vi "TurnAngleOperationOpenLoop.vi"(7 "RobotDriveRef in":T1={"RobotDriveDevRef"={"DevStatus"={"status"=FALSE, "code"=0, "source"=""}, "Motors[]"=[], "Square Inputs"=FALSE, "Max Output"=0.0}, "Control Mode"=enum."Percent VBus", "Motor Settings"={"Wheel Radius"=0.0, "Encoder Ticks Per Rev"=0.0, "Gear Ratio"=0.0, "ClimbRev"=0.0}, "Default Control Mode"=enum."Unchanged / Invalid", "Speed Mag"=0.0}, 8 "error in (no error)":errorcluster, 9 "SubSystem Data":T10, 10 "Control Mode":T8, 11 "Command Loop Data":cluster{"Start Time (ms)":u32, "Iterations":i32}) -> (0 "error out":errorcluster, 1 "Left Motor Value":dbl, 2 "RobotDriveRef out":T1={"RobotDriveDevRef"={"DevStatus"={"status"=FALSE, "code"=0, "source"=""}, "Motors[]"=[], "Square Inputs"=FALSE, "Max Output"=0.0}, "Control Mode"=enum."Percent VBus", "Motor Settings"={"Wheel Radius"=0.0, "Encoder Ticks Per Rev"=0.0, "Gear Ratio"=0.0, "ClimbRev"=0.0}, "Default Control Mode"=enum."Unchanged / Invalid", "Speed Mag"=0.0}, 3 "Wait Time":dbl, 4 "Waveform Chart":cluster{"Angle To Turn out":dbl, "Yaw":dbl}(graph), 5 "Finished":bool, 6 "Right Motor Value":dbl)   [LabVIEW 2015]
uses:
  Drive Setpoints.ctl
  Drive Operations.ctl
  Advanced Drive VIs/RobotDrive Type Def.ctl
  <vilib>/Rock Robotics/WPI/MotorControl/WPI_MotorControlDeviceRef.ctl
  <vilib>/Rock Robotics/WPI/MotorControl/WPI_MotorControlType.ctl
  <vilib>/Rock Robotics/SystemInterfaces/DIO/FPGA_DIOPWMChannel.ctl
  <vilib>/Rock Robotics/WPI/PWM/WPI_PWMDeadband.ctl
  <vilib>/Rock Robotics/WPI/CAN/Jaguar/SubVIs/WPI_CANJaguar_ControlMode.ctl
  <vilib>/Rock Robotics/WPI/CAN/TalonSRX/WPI_CANTalonSRX_APIControlMode.ctl
  Advanced Drive VIs/Drive Motor Settings.ctl
  NavX/NavX Global.vi
  NavX/Library/navX Library v2.lvlib
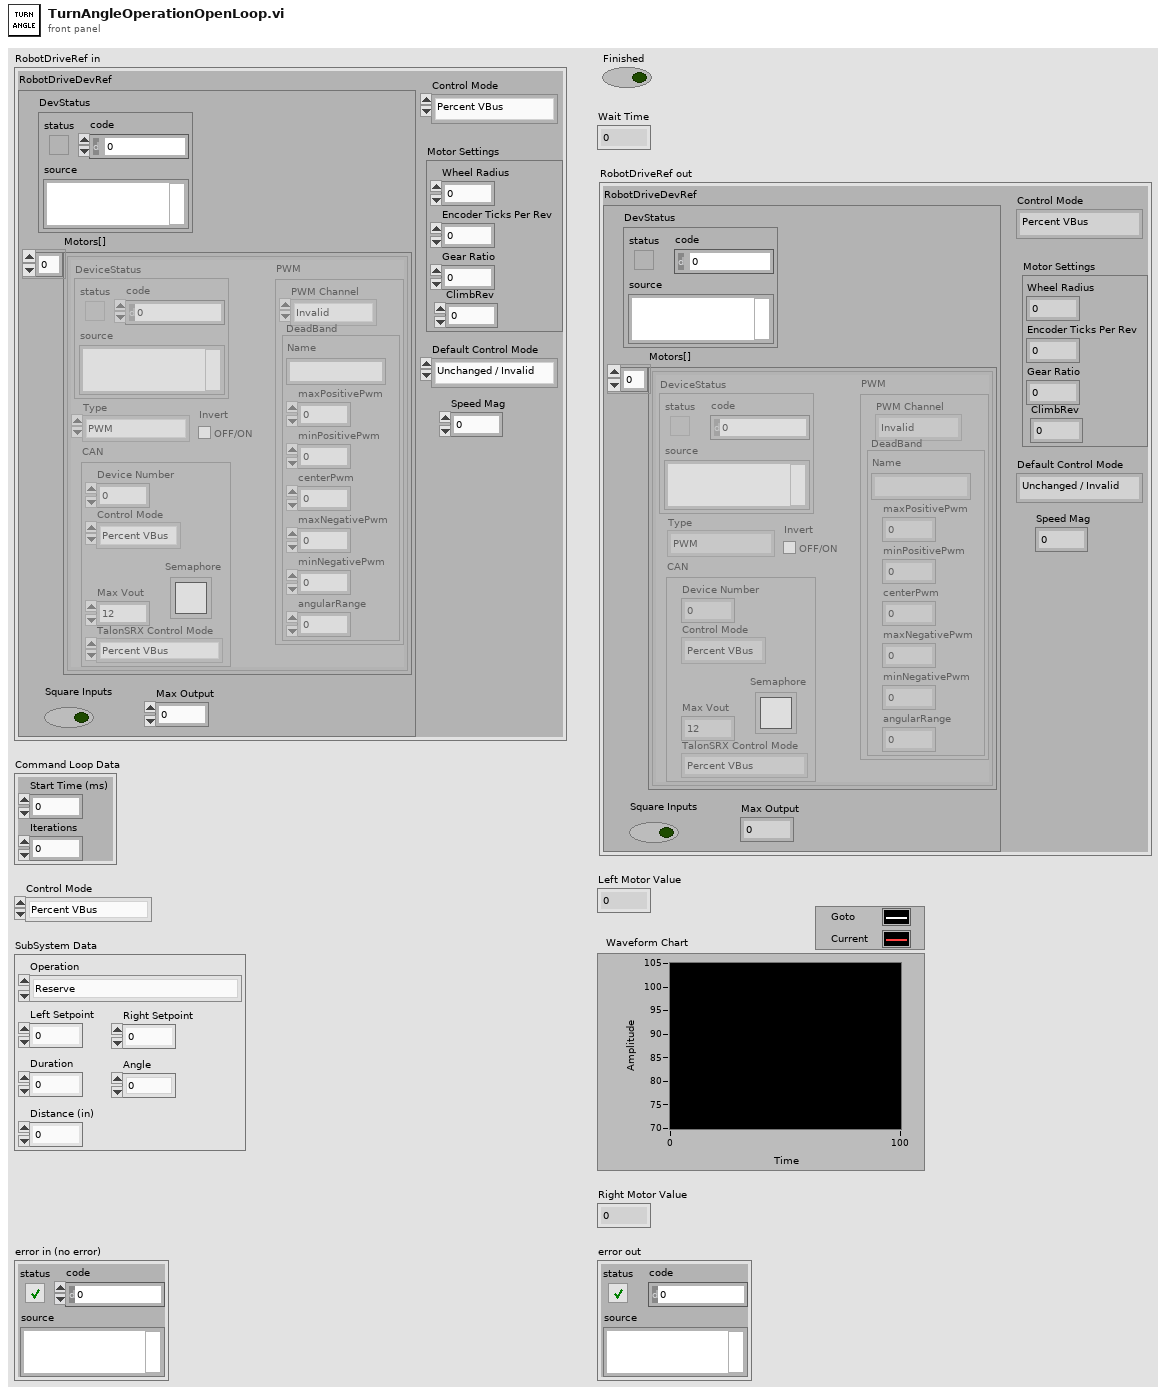
[diagram p1: front panel]
types:
  T1 = typedef "RobotDrive Type Def.ctl" = cluster{"RobotDriveDevRef":cluster{"DevStatus":errorcluster, "Motors[]":T2[], "Square Inputs":bool, "Max Output":dbl}, "Control Mode":T8, "Motor Settings":T9, "Default Control Mode":T8, "Speed Mag":dbl}
  T2 = typedef "WPI_MotorControlDeviceRef.ctl" = cluster{"DeviceStatus":errorcluster, "Type":T3, "PWM":cluster{"PWM Channel":T4, "DeadBand":T5}, "CAN":cluster{"Device Number":u8, "Control Mode":T6, "Semaphore":T7, "Max Vout":dbl, "TalonSRX Control Mode":T8}, "Invert":bool}
  T3 = typedef "WPI_MotorControlType.ctl" = enum16{"PWM", "CAN", "CANTalonSRX"}
  T4 = typedef "FPGA_DIOPWMChannel.ctl" = enum8{"PWM 0", "PWM 1", "PWM 2", "PWM 3", "PWM 4", "PWM 5", "PWM 6", "PWM 7", "PWM 8", "PWM 9", "PWM MXP 0", "PWM MXP 1", "PWM MXP 2", "PWM MXP 3", "PWM MXP 4", "PWM MXP 5", "PWM MXP 6", "PWM MXP 7", "PWM MXP 8", "PWM MXP 9", "Invalid"}
  T5 = typedef "WPI_PWMDeadband.ctl" = cluster{"Name":string, "maxPositivePwm":i32, "minPositivePwm":i32, "centerPwm":i32, "maxNegativePwm":i32, "minNegativePwm":i32, "angularRange":u16}
  T6 = typedef "WPI_CANJaguar_ControlMode.ctl" = enum8{"Percent VBus", "Current", "Speed", "Position", "Voltage"}
  T7 = typedef "Semaphore RefNum" = refnum<k1>
  T8 = typedef "WPI_CANTalonSRX_APIControlMode.ctl" = enum8{"Percent VBus", "Speed", "Position", "Slave", "Unchanged / Invalid", "Voltage Compensation", "Current", "Motion Profile"}
  T9 = typedef "Drive Motor Settings.ctl" = cluster{"Wheel Radius":dbl, "Encoder Ticks Per Rev":dbl, "Gear Ratio":dbl, "ClimbRev":dbl}
  T10 = typedef "Drive Setpoints.ctl" = cluster{"Operation":T11, "Left Setpoint":dbl, "Right Setpoint":dbl, "Duration":dbl, "Angle":dbl, "Distance (in)":dbl}
  T11 = typedef "Drive Operations.ctl" = enum16{"Reserve", "Read Current", "Immediate", "Drive for Time", "Drive for Distance", "Turn Degrees"}
  T12 = cluster{"Yaw":dbl, "Roll":dbl, "Pitch":dbl, "Heading":dbl, "Fused Heading":dbl}
  T13 = typedef "navX Library v2.lvlib/Z900_navX_DeviceTypeDef.ctl" = cluster{"Interface":cluster{"Protocol":T14, "Update Rate (4Hz-60Hz)":u8, "navX Open TypeDef":variant}, "Notify Packet":refnum<notifier>, "Loop VI Refnum":refnum<vi>, "Ready to Close Occurrence Refnum":refnum<k4>}
  T14 = typedef "navX Library v2.lvlib/Z900_navX_ProtocolTypeDef.ctl" = enum16{"SERIAL", "I2C", "SPI"}
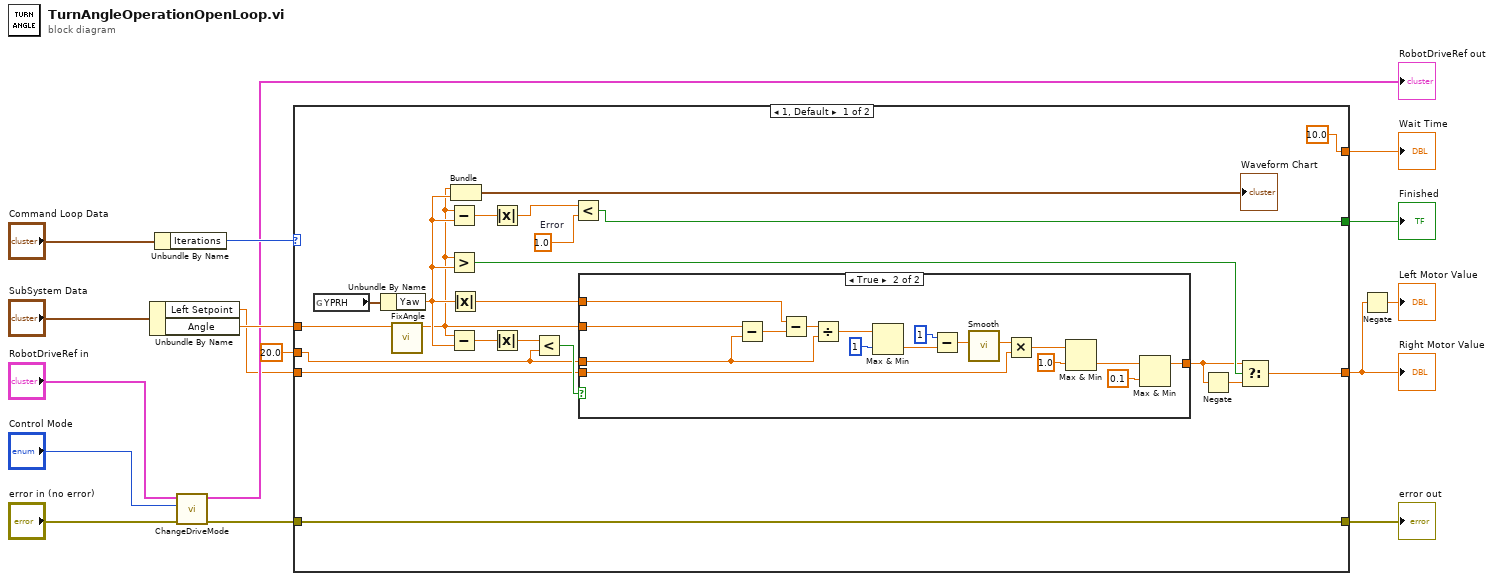
[diagram p0: block diagram]
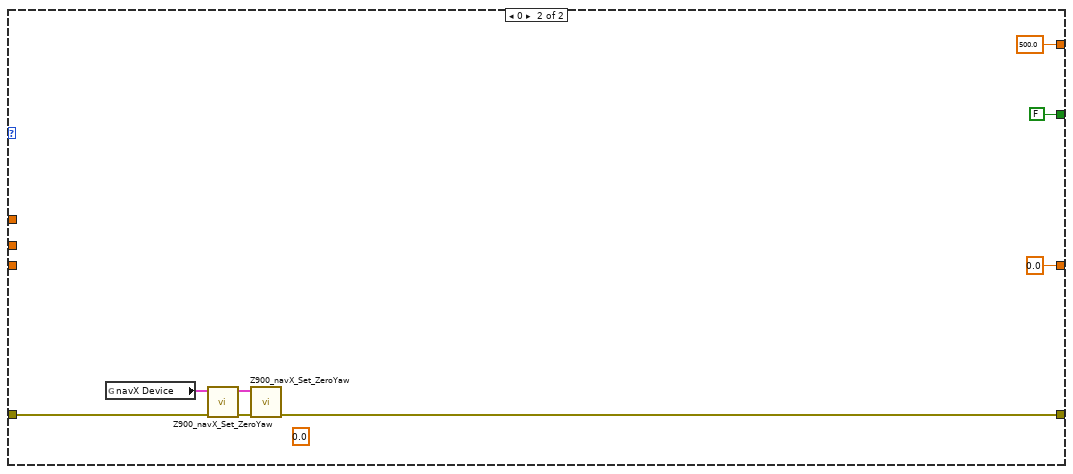
[diagram p3: hidden frame]
diagram:
  n1 = Unbundle By Name("SubSystem Data") -> ("Left Setpoint"=w4:dbl, "Angle"=w16:dbl)
  n2 = Unbundle By Name("Command Loop Data") -> ("Iterations"=w13:i32)
  n3 = call "ChangeDriveMode.vi"("error in (no error)"="error in (no error)", "Control Mode"="Control Mode", "RobotDriveRef"="RobotDriveRef in") -> ("error out"=w6:errorcluster, "RobotDriveRef Out"=→"RobotDriveRef out":T1)  [unwired: 7 in]
  n4 = case shown="1, Default" w13 {
    tunnel: [w26 0.0 ("Left Motor Value")] -> w2
    tunnel: w16 -> [w33 _]
    tunnel: [w32 FALSE] -> w14
    tunnel: [10.0 500.0] -> w11
    tunnel: w6 -> [w30 w57]
    tunnel: [w30 w56] -> w5
    tunnel: w4 -> [w17 _]
    tunnel: 20.0 -> [w18 _]
    frame 1, Default {
      w34 = 1.0  # Error
      n5 = global read "NavX Global.vi" "YPRH"() -> (w37:T12)
      n6 = Unbundle By Name(w37) -> ("Yaw"=w21:dbl)
      n7 = call "FixAngle.vi"("Angle To Turn in"=w33) -> ("Angle To Turn out"=w19:dbl)  [unwired: 10 in]
      n8 = Subtract(x=w19, y=w21) -> (x-y=w36:dbl)
      n9 = Greater?(x=w19, y=w21) -> (0:w29:bool)
      n10 = Subtract(x=w19, y=w21) -> (x-y=w25:dbl)
      n11 = Absolute Value(x=w21) -> (abs(x)=w20:dbl)
      n12 = Bundle("Angle To Turn out"=w19, "Yaw"=w21) -> (→"Waveform Chart":cluster{"Angle To Turn out":dbl, "Yaw":dbl})  [unwired: 1 in]
      n13 = Absolute Value(x=w36) -> (abs(x)=w35:dbl)
      n14 = Absolute Value(x=w25) -> (abs(x)=w24:dbl)
      n15 = Less?(x=w24, y=w18) -> (x < y?=w23:bool)
      n16 = Less?(x=w35, y=w34) -> (x < y?=w32:bool)
      n17 = case shown="True" w23 {
        tunnel: w17 -> [w38 w42]
        tunnel: [w38 w39] -> w22
        tunnel: w20 -> [_ w45]
        tunnel: w19 -> [_ w44]
        tunnel: w18 -> [_ w43]
        frame False {
        }
        frame True {
          n18 = Subtract(x=w44, y=w43) -> (x-y=w55:dbl)
          n19 = Subtract(x=w45, y=w55) -> (x-y=w53:dbl)
          n20 = Divide(x=w53, y=w43) -> (x/y=w49:dbl)
          n21 = Max & Min(x=w49, y=1) -> (min(x,y)=w48:dbl)  [unwired: 1 out]
          n22 = Subtract(x=1, y=w48) -> (x-y=w51:dbl)
          n23 = call "Smooth.vi"("x"=w51) -> ("y"=w41:dbl)  [unwired: 10 in]
          n24 = Multiply(x=w41, y=w42) -> (x*y=w40:dbl)
          n25 = Max & Min(x=w40, y=1.0) -> (min(x,y)=w47:dbl)  [unwired: 1 out]
          n26 = Max & Min(x=w47, y=0.1) -> (max(x,y)=w39:dbl)  [unwired: 1 out]
        }
      }
      n27 = Negate(x=w22) -> (-x=w28:dbl)
      n28 = Select(t=w22, s=w29, f=w28) -> (s? t:f=w26:dbl)
    }
    frame 0 {
      (unwired) 0.0 ("Right Motor Value")
      n29 = global read "NavX Global.vi" "navX Device"() -> (w60:T13)
      n30 = call "Z900_navX_Set_ZeroYaw.vi"("error in (no error)"=w57, "navX Device"=w60) -> ("error out"=w58:errorcluster, "navX Device"=w59:T13)  [unwired: 8 in]
      n31 = call "Z900_navX_Set_ZeroYaw.vi"("error in (no error)"=w58, "navX Device"=w59) -> ("error out"=w56:errorcluster)  [unwired: 8 in, 1 out]
    }
  }
  "Finished" <- w14
  "error out" <- w5
  "Wait Time" <- w11
  "Right Motor Value" <- w2
  n32 = Negate(x=w2) -> (-x=→"Left Motor Value":dbl)
